vi "Read Homing.vi"(8 "error in (no error)":errorcluster, 11 "FW Arduino Control in":refnum<class "FW Arduino Control.lvclass">) -> (0 "error out":errorcluster, 2 "Homing":variant, 3 "FW Arduino Control out":refnum<class "FW Arduino Control.lvclass">)   [LabVIEW 2021, in "FW Arduino Control.lvclass"]
uses:
  FW Arduino Control.lvclass
  FW Arduino Control.lvclass/FW Arduino Control.ctl
  Filter Wheel Object/Filter Wheel.lvclass
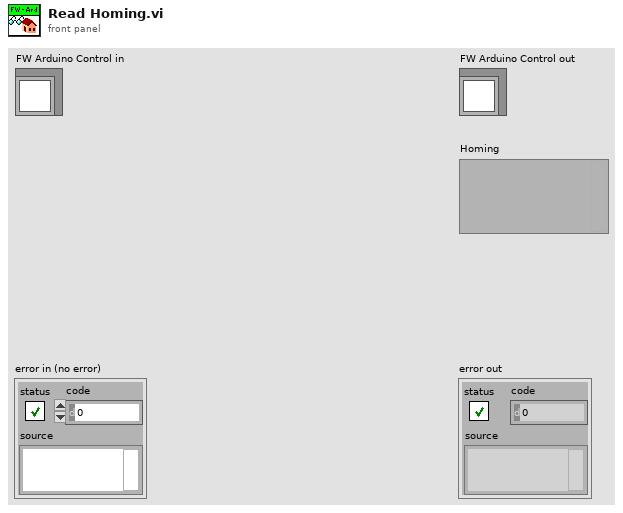
[diagram p1: front panel]
types:
  T1 = typedef "Filter Wheel Arduino Homing cluster.ctl" = cluster{"Direction (F: CW)":bool, "Speed":i32, "Accel":i32, "Min Distance":i32, "Short Leg":i32, "Error Cnts":i32}
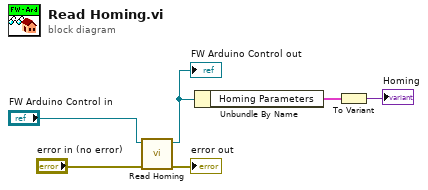
[diagram p0: block diagram]
diagram:
  n1 = call-parent "Read Homing.vi"("error in (no error)"="error in (no error)", "Filter Wheel in"="FW Arduino Control in") -> ("error out"=→"error out":errorcluster, "Filter Wheel out"=w3:refnum<class "FW Arduino Control.lvclass">)  [unwired: 7 in, 1 out]
  "FW Arduino Control out" <- w3
  n2 = Unbundle By Name(w3) -> ("Homing Parameters"=w2:T1)
  n3 = To Variant(anything=w2) -> (Variant=→"Homing":variant)
